vi "Rotate Flip Layer.vi"(8 "error in (no error)":errorcluster, 9 "Rotate":bool, 10 "Reset origin?":bool, 11 "Layer in":refnum<class "Layer.lvclass">) -> (0 "error out":errorcluster, 3 "Layer out":refnum<class "Layer.lvclass">)   [LabVIEW 2020, in "LabVIEW Icon API.lvlib"]
doc: "Rotate or Flip the User Layer glyph."
uses:
  LabVIEW Icon API.lvlib
  lv_icon/Classes/Layer/Layer.lvclass
  resource/plugins/lv_icon.lvlib
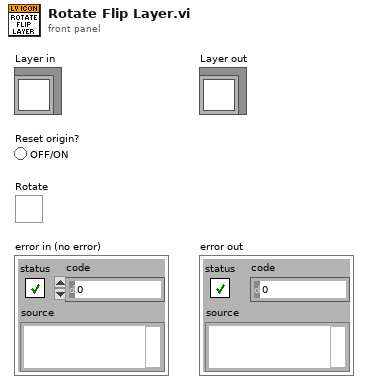
[diagram p1: front panel]
types:
  T1 = cluster{"left":i16, "top":i16, "right":i16, "bottom":i16}
  T2 = typedef "Layer.ctl" = cluster{"LayerIcon":picture, "LayerName":string, "Opacity":u8, "Visibility?":bool}
  T3 = typedef "LVPoint32TypeDef.ctl" = cluster{"Horizontal":i32, "Vertical":i32}
  T4 = cluster{"left":i16, "top":i16, "bottom":i16, "right":i16}
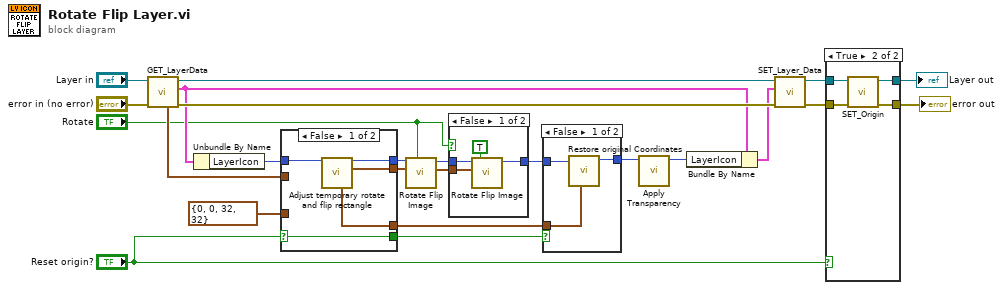
[diagram p0: block diagram]
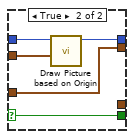
[diagram p4: hidden frame]
diagram:
  n1 = call-dynamic "GET_LayerData.vi"("error in (no error)"="error in (no error)", "Layer.lvclass in"="Layer in") -> ("error out"=w22:errorcluster, "Data"=w5:T2, "Layer.lvclass out"=w3:refnum<class "Layer.lvclass">, "Origin"=w19:T3)  [unwired: 6 out]
  n2 = Unbundle By Name(w5) -> ("LayerIcon"=w18:picture)
  n3 = case shown="False" "Reset origin?" {
    selector: "Reset origin?" -> [w25 w34]
    tunnel: w18 -> [w29 w32]
    tunnel: [w28 w31] -> w9
    tunnel: [w27 w33] -> w10
    tunnel: [w26 _] -> w13
    tunnel: [w25 w34] -> w14
    tunnel: T1 {"left"=0, "top"=0, "right"=32, "bottom"=32} ("rect") -> [_ w33]
    tunnel: w19 -> [_ w30]
    frame False {
      n4 = call "Adjust temporary rotate and flip rectangle.vi"("Pic in"=w29) -> ("temp subset rect"=w27:cluster{i32, i32, "b-a":i32, "b-a":i32}, "Pic out"=w28:picture, "true subset rect"=w26:T1)  [unwired: 8 out]
    }
    frame True {
      n5 = call "Draw Picture based on Origin.vi"("Origin"=w30, "LayerIcon in"=w32) -> ("LayerIcon out"=w31:picture)  [unwired: 1 in, 8 out]
    }
  }
  n6 = call "Rotate Flip Image.vi"("Rotate?"="Rotate", "rect"=w10, "Temp Icon In"=w9) -> ("rect out"=w8:T4, "Temp Icon Out"=w7:picture)  [unwired: 7 out]
  n7 = case shown="False" "Rotate" {
    tunnel: w7 -> [w38 w39]
    tunnel: [w37 w39] -> w11
    tunnel: w8 -> [w35 _]
    frame False {
      n8 = call "Rotate Flip Image.vi"("Rotate?"=TRUE, "rect"=w35, "Temp Icon In"=w38) -> ("Temp Icon Out"=w37:picture)  [unwired: 8 out]
    }
    frame True {
    }
  }
  n9 = case shown="False" w14 {
    tunnel: w11 -> [w42 w43]
    tunnel: [w41 w43] -> w12
    tunnel: w13 -> [w40 _]
    frame False {
      n10 = call "Restore original Coordinates.vi"("temp size in"=w40, "Pic in"=w42) -> ("Pic out"=w41:picture)  [unwired: 9 out]
    }
    frame True {
    }
  }
  n11 = call "Apply Transparency.vi"("in"=w12) -> ("out"=w2:picture)  [unwired: 10 in]
  n12 = Bundle By Name(cluster=w5, "LayerIcon"=w2) -> (w4:T2)
  n13 = call-dynamic "SET_Layer_Data.vi"("error in (no error)"=w22, "Data"=w4, "Layer.lvclass in"=w3) -> ("error out"=w23:errorcluster, "Layer.lvclass out"=w16:refnum<class "Layer.lvclass">)  [unwired: 1 in, 6 out]
  n14 = case shown="True" "Reset origin?" {
    tunnel: w23 -> [w45 w49]
    tunnel: w16 -> [w44 w47]
    tunnel: [w44 w46] -> w17
    tunnel: [w45 w48] -> w24
    frame False {
    }
    frame True {
      n15 = call-dynamic "SET_Origin.vi"("error in"=w49, "Layer.lvclass in"=w47) -> ("error out"=w48:errorcluster, "Layer.lvclass out"=w46:refnum<class "Layer.lvclass">)  [unwired: 8 in]
    }
  }
  "error out" <- w24
  "Layer out" <- w17
